vi "MasterControl.vi"() -> ()   [LabVIEW 2012]
uses:
  VI State Control.ctl
  TMC/Set Parameter.ctl
  LabView VI's/Source Mirror Manipulator/Axis.ctl
  SMC VIs - Pollux/SMC SubVIs/SMC_SubVIs.llb/SMC Paras.ctl
  SMC VIs - Pollux/SMC SubVIs/SMC_SubVIs.llb/VENUSNr.ctl
  SMC VIs - Pollux/SubVIs/JS_Comm.llb/Comm_Paras.ctl
  SMC VIs - Pollux/SubVIs/JS_Comm.llb/Comm_Method.ctl
panel:
  out "Diode 1":string
  out "Diode 3":string
  out "Diode 2":string
  in  "Time Delay":u32
  in  "File Path for Data Log":path=path "C:/Users/user/Desktop/labviewMove/stats/stats_00-00-00.txt"
  out "Error":bool
  out "VI Status":bool
  in  "Anode Control":enum16{"1", "2", "3", "4", "5", "6"}(ring)
  out "Axis Information":string
  in  "Axis Positions":T1
  out "VI State Control":T2
  out "Source Mirror Position (mm)":dbl(slide) scale=0.0..50.0 scale format="%#.6g"
  in  "Voltage Value":dbl
  in  "Set Source Voltage":bool
  out "Current (mA)":dbl
  out "Source Voltage":dbl
  out "Logging Indicator":bool
  in  "Source Voltage Control":bool
  out "Limit A":bool
  out "Limit B":bool
  out "Home":bool
  in  "Main Axis Control":T3(ring)
  out "Anode :":u32(knob) scale=1.0..6.0
  in  "Target":dbl
  out "Current Position:":dbl
  in  "Absolute Position Value":dbl
  in  "Index +/- Value":dbl
  in  "Stop Program":bool
  in  "Abort Motion":bool
  in  "Stop Motion Softly":bool
  in  "Move to Absolute Positon":bool
  in  "Position Index +/-":bool
  in  "Reset Position to Target":bool
  in  "Go To Home Position":bool
  # "--  Master Control  --"
  # "sec"
  # "Data Logging Control"
  # "Keep file type as a '.txt' file"
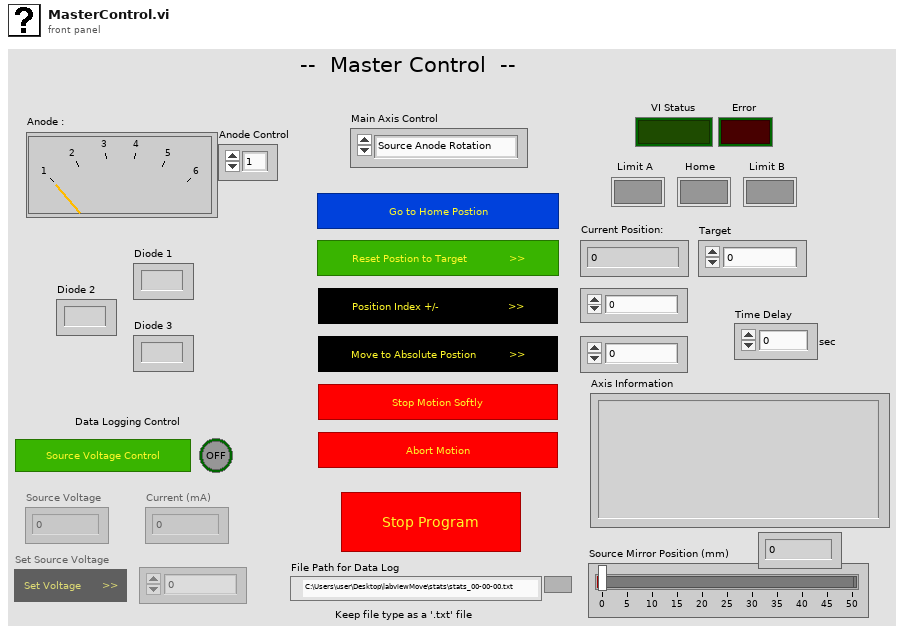
[diagram p1: front panel]
types:
  T1 = cluster{"Source Anode Rotation (P)":dbl, "Aperture Translation (P)":dbl, "Grating Translation (P)":dbl, "Grating Vertical (P)":dbl, "Grating Rotation (P)":dbl, "Polarization Angle (P)":dbl, "Source Mirror Translation (P)":dbl, "Source Mirror Rotation (P)":dbl, "Camera Translation (P)":dbl, "Camera Vertical (P) ":dbl, "Detector Mirror Rotation (P)":dbl}
  T2 = typedef "VI State Control.ctl" = enum16{"Initialization", "Wait for Command", "Add New State Here"}
  T3 = enum16{"Source Anode Rotation", "Aperture Translation", "Grating Translation", "Grating Vertical", "Grating Rotation", "Polarization Angle", "Source Mirror Translation", "Source Mirror Rotation", "Camera Translation", "Camera Vertical", "Detector Mirror Rotation"}
  T4 = enum16{"open", "replace", "create", "open or create", "replace or create", "replace or create with confirmation"}
  T5 = typedef "Axis.ctl" = enum16{"Translation", "Rotation"}
  T6 = typedef "Set Parameter.ctl" = enum16{"Acceleration (A)", "Baud Rate (BD)", "Counter 1 (C1)", "Counter 2 (C2)", "Control C Software Reset (CE)", "Check Sum Enable (CK)", "Clock Mode (CM)", "Clock Mode Ratio (CR)", "Clock Mode Out Step Width (CW)", "Deceleration (D)", "Digital Filtering, Input 1 (D1)", "Digital Filtering, Input 2 (D2)", "Digital Filtering, Input 3 (D3)", "Digital Filtering, Input 4 (D4)", "Digital Filtering, Input 5 (D5)", "Digital Filtering, Input 9 (D9)", "Digital Filtering, Input 10 (D10)", "Digital Filtering, Input 11 (D11)", "Digital Filtering, Input 12 (D12)", "Deadband (DB)", "Decrement Variable (DC)", "Enable/Disable Drive (DE)", "Device Name (DN)", "End Program Execution (E)", "Encoder Function Enable (EE)", "Encoder Lines (EL)", "Echo Mode (EM)", "Escape (ES)", "Execute Program at Address (EX)", "Hold (H)", "Hold Current (HC)", "Hold Current Delay Time (HI)", "Home to Encoder Index (HM)", "Home to Home Switch (HT)", "Increment Variable (IC)", "Initialize Parameters to NVM (IP)", "Input into Variable (IV)", "Jog Enable (JE)", "Limit Stop Mode (LM)", "Move Absolute (MA)", "Move Relative (MR)", "MicroStepping Select (MS)", "Motor Settling Delay Time (MT)", "Output 1 (O1)", "Output 2 (O2)", "Output 3 (O3)", "Output 4 (O4)", "Output 9 (O9)", "Output 10 (O10)", "Output 11 (O11)", "Output 12 (O12)", "Output High Byte (9-12) (OH)", "Output Low Byte (1-4) (OL)", "Output Total (1-4 and 9-12) (OT)", "Position Maintenance (PM)", "Party Mode (PY)", "Register 1 (R1)", "Register 2 (R2)", "Register 3 (R3)", "Register 4 (R4)", "Run Current (RC)", "Stall Factor (SF)", "Slew (SL)", "Stall Mode Set (SM)", "Upgrade Firmware (UG)", "Velocity Initial (VI)", "Velocity Maximum (VM)"}
  T7 = typedef "Comm_Paras.ctl" = cluster{"Comm Method":T8, "IP Address":string, "Remote Port":u16, "GPIB Address":string, "VISA Resource Name":refnum<visa-resource-name>, "Visa Baud Rate":u32, "Visa Serial":bool}
  T8 = typedef "Comm_Method.ctl" = enum16{"TCPIP", "GPIB", "VISA"}
  T9 = typedef "SMC Paras.ctl" = cluster{"VENUS Language":T10, "Number of Axis":u8, "Controller Nr":u8, "Simulation":bool}
  T10 = typedef "VENUSNr.ctl" = enum16{"VENUS 2", "VENUS 1"}
  T11 = enum8{"Enabled", "Disabled", "Disabled and Grayed Out"}
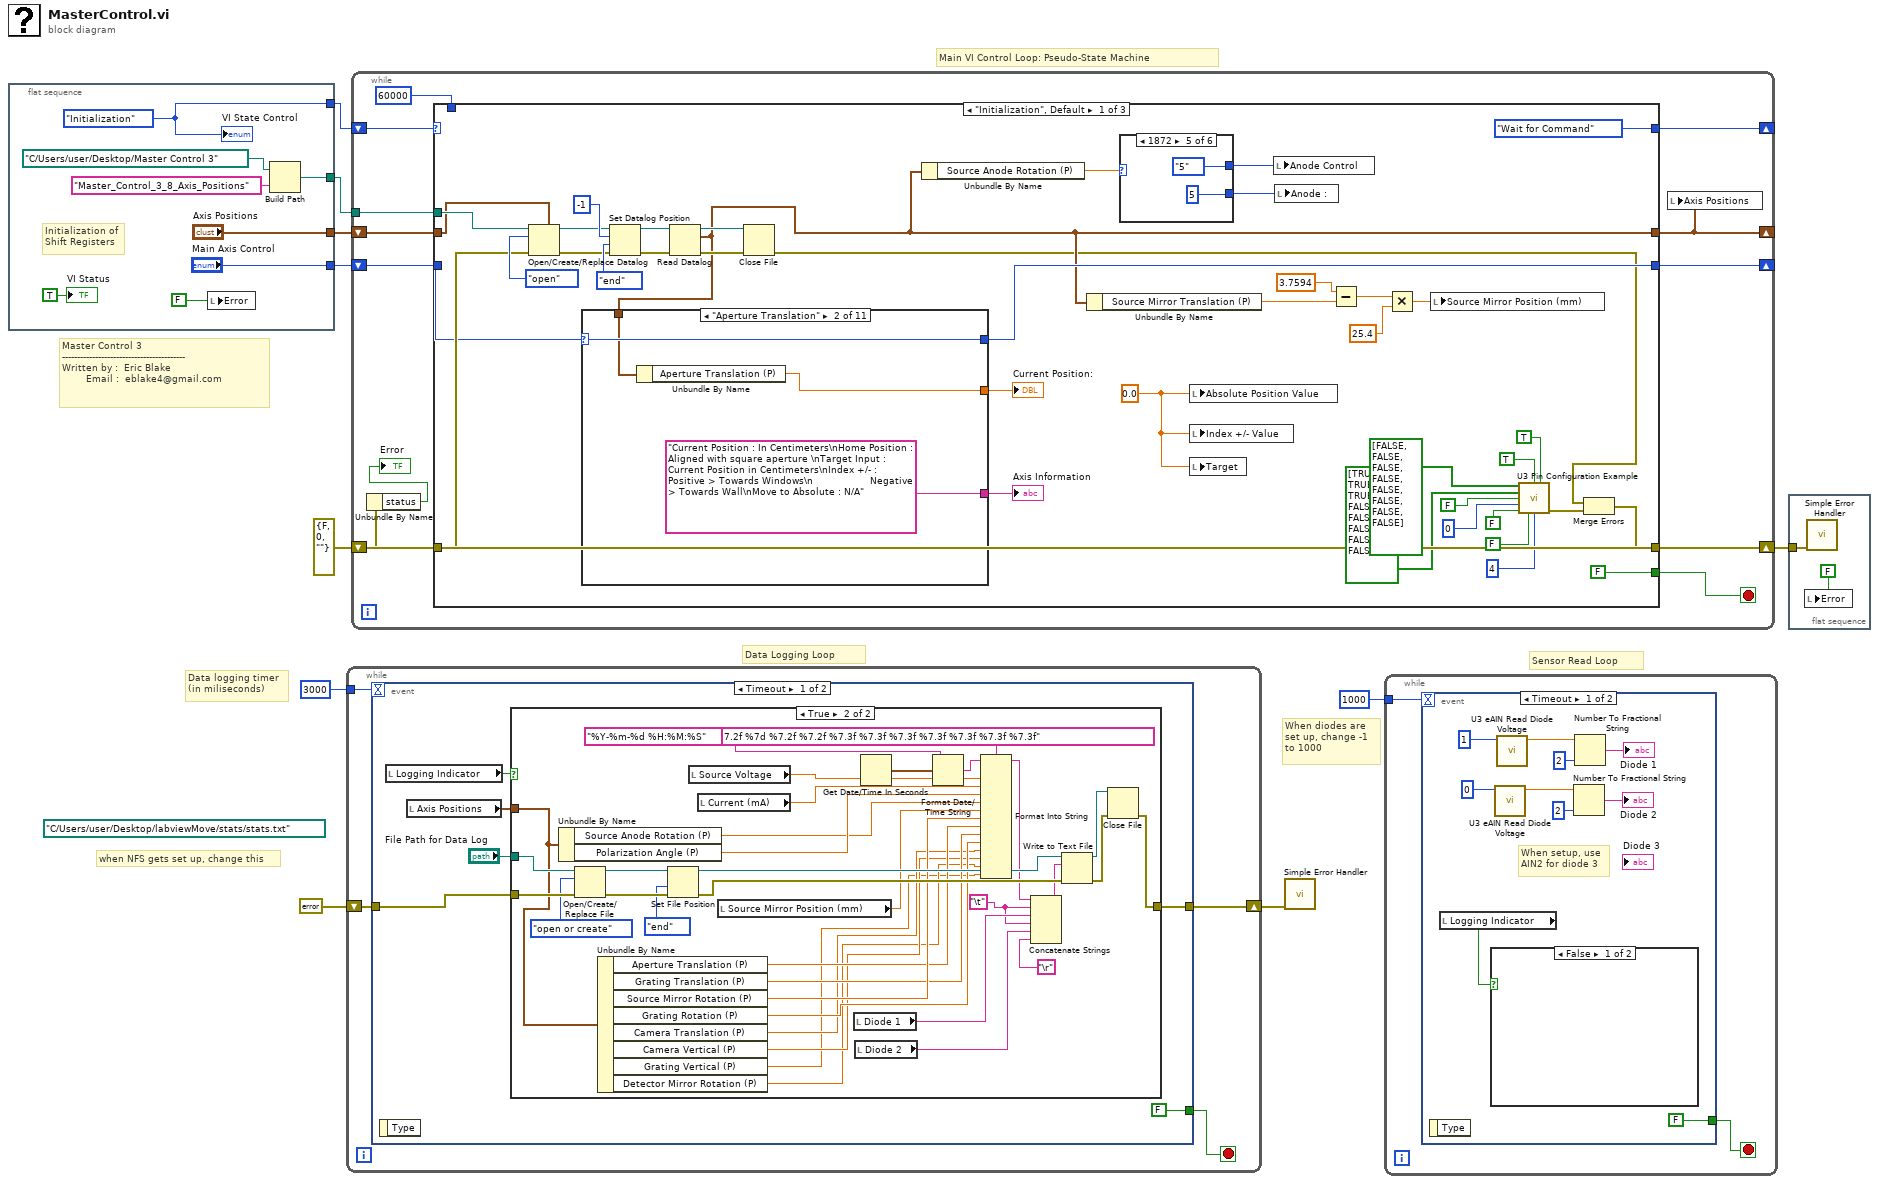
[diagram p0: block diagram]
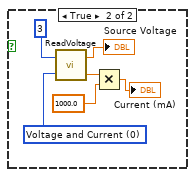
[diagram p2: hidden frame]
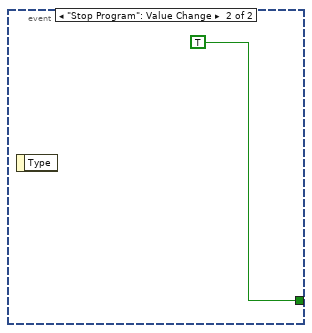
[diagram p3: hidden frame]
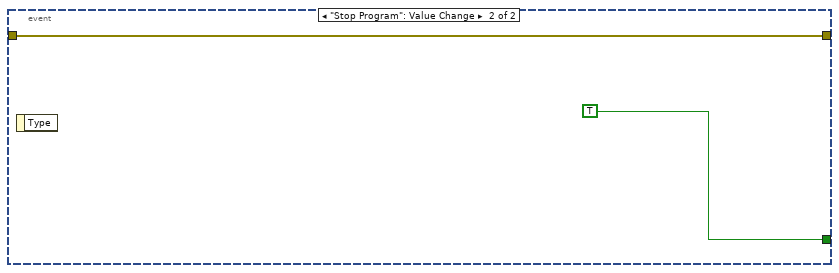
[diagram p5: hidden frame]
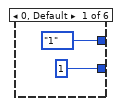
[diagram p6: hidden frame]
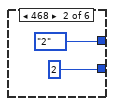
[diagram p7: hidden frame]
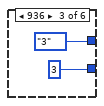
[diagram p8: hidden frame]
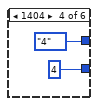
[diagram p9: hidden frame]
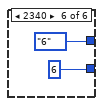
[diagram p10: hidden frame]
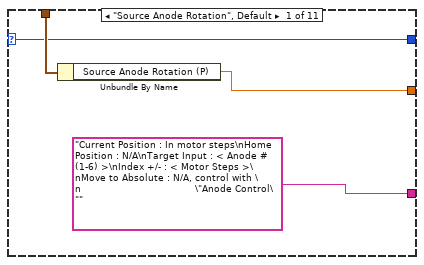
[diagram p11: hidden frame]
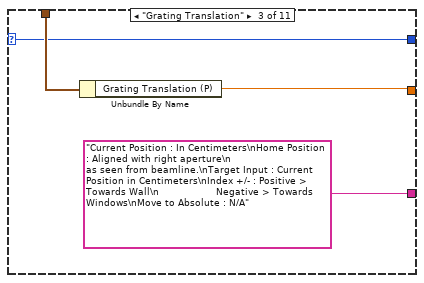
[diagram p12: hidden frame]
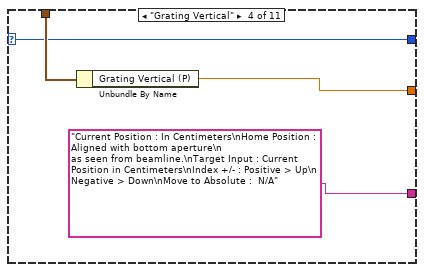
[diagram p13: hidden frame]
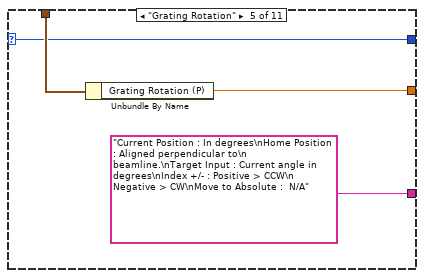
[diagram p14: hidden frame]
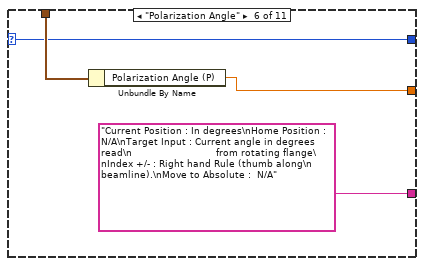
[diagram p15: hidden frame]
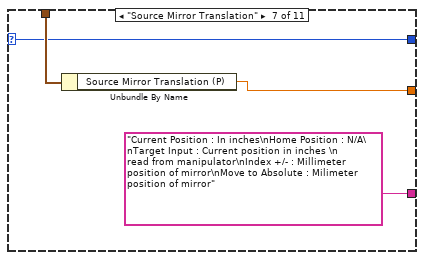
[diagram p16: hidden frame]
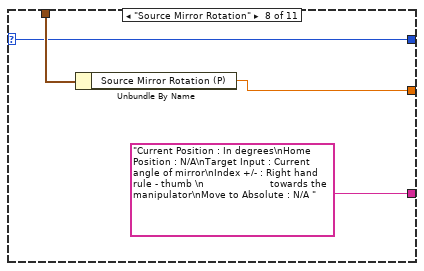
[diagram p17: hidden frame]
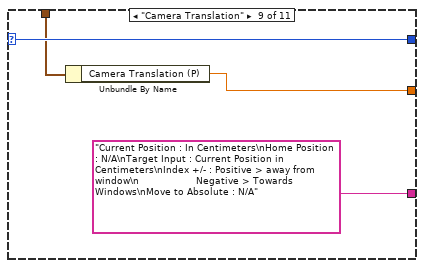
[diagram p18: hidden frame]
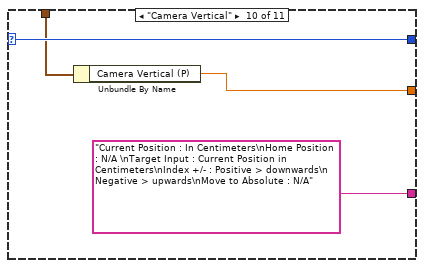
[diagram p19: hidden frame]
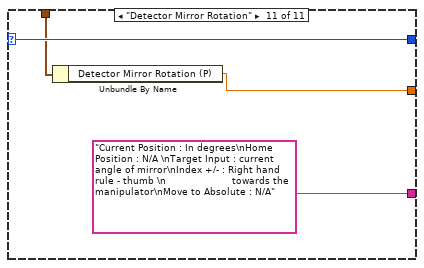
[diagram p20: hidden frame]
diagram:
  (unwired) path "C:/Users/user/Desktop/labviewMove/stats/stats.txt" ("file path (use dialog)")
  # "Master Control 3\n-----------------------------------------\nWritten by :  Eric Blake\n        Email :  eblake4@gmail.com"
  # "when NFS gets set up, change this"
  # "When diodes are \nset up, change -1 \nto 1000"
  # "Sensor Read Loop"
  # "Main VI Control Loop: Pseudo-State Machine"
  # "Data Logging Loop"
  # "Data logging timer\n(in miliseconds)"
  n1 = flat-sequence {
    tunnel: [w18] -> w10
    tunnel: [w15] -> w8
    tunnel: ["Main Axis Control"] -> w7
    tunnel: ["Axis Positions"] -> w6
    frame #0 {
      w18 = VI_State_Control."Initialization" ("VI State Control")
      # "Initialization of\nShift Registers"
      n2 = local write "Error"(FALSE) -> ()
      n3 = Build Path(base path=path "C:/Users/user/Desktop/Master Control 3", name or relative path="Master_Control_3_8_Axis_Positions") -> (appended path=w15:path)
      "VI State Control" <- w18
      "VI Status" <- TRUE ("VI on")
    }
  }
  n4 = while {
    tunnel: 3000 -> [w22]
    shift-right: [w19] -> w3
    shift-left: errorcluster {"status"=FALSE, "code"=0, "source"=""} ("error out") -> [w20]
    stop <- w21 stop-if-true
    n5 = event shown="[0] Timeout" {
      selector: _ -> [_ _]
      dyn-events: _ -> [_ _]
      timeout: w22 -> [_ _]
      tunnel: [FALSE TRUE] -> w21
      tunnel: [w25 w65] -> w19
      tunnel: w20 -> [w24 w65]
      event Timeout {
        n6 = event-data() -> ()  [unwired: 1 in, 1 out]
        n7 = local read "Logging Indicator"() -> (w26:bool)
        n8 = local read "Axis Positions"() -> (w27:T1)
        n9 = case shown="True" w26 {
          tunnel: w27 -> [_ w45]
          tunnel: [w29 w52] -> w25
          tunnel: w24 -> [w29 w51]
          tunnel: "File Path for Data Log" -> [_ w48]
          frame False {
          }
          frame True {
            w36 = "\t"
            n10 = Unbundle By Name(w45) -> ("Source Anode Rotation (P)"=w53:dbl, "Polarization Angle (P)"=w57:dbl)
            n11 = Open/Create/Replace File(file path (use dialog)=w48, error in=w51, operation (0:open)=T4."open or create") -> (refnum out=w63:refnum<file>, error out=w64:errorcluster)  [unwired: 4 out]
            n12 = Unbundle By Name(w45) -> ("Aperture Translation (P)"=w42:dbl, "Grating Translation (P)"=w41:dbl, "Source Mirror Rotation (P)"=w43:dbl, "Grating Rotation (P)"=w34:dbl, "Camera Translation (P)"=w33:dbl, "Camera Vertical (P)"=w32:dbl, "Grating Vertical (P)"=w30:dbl, "Detector Mirror Rotation (P)"=w31:dbl)
            n13 = Set File Position(refnum=w63, from (0:start)=enum16{"start", "end", "current"}."end", error in=w64) -> (refnum out=w56:refnum<file>, error out=w50:errorcluster)  [unwired: 1 out]
            n14 = local read "Source Voltage"() -> (w46:dbl)
            n15 = local read "Current (mA)"() -> (w47:dbl)
            n16 = local read "Source Mirror Position (mm)"() -> (w49:dbl)
            n17 = local read "Diode 1"() -> (w37:string)
            n18 = local read "Diode 2"() -> (w35:string)
            n19 = Get Date/Time In Seconds() -> (seconds since 1Jan1904=w61:timestamp)
            n20 = Format Date/Time String(time format string (%c)="%Y-%m-%d %H:%M:%S", seconds (now)=w61) -> (date/time string=w59:string)  [unwired: 1 out]
            n21 = Format Into String(format string=" %7.1f %7.4f %+7.2f %7d %7.2f %7.2f %7.3f %7.3f %7.3f %7.3f %7.3f %7.3f %7.3f", initial string=w59, w46, w47, w57, w53, w49, w43, w42, w41, w34, w33, w32, w31, w30) -> (resulting string=w40:string)  [unwired: 1 in, 1 out]
            n22 = Concatenate Strings(w40, w36, w37, w36, w35, "\r") -> (w39:string)
            n23 = Write to Text File(file (use dialog)=w56, text=w39, error in=w50) -> (refnum out=w55:refnum<file>, error out=w54:errorcluster)  [unwired: 2 out]
            n24 = Close File(refnum=w55, error in=w54) -> (error out=w52:errorcluster)  [unwired: 1 out]
          }
        }
      }
      event "Stop Program": Value Change {
        n25 = event-data() -> ()  [unwired: 1 in, 1 out]
      }
    }
  }
  n26 = while {
    tunnel: w8 -> [w76]
    shift-right: [w77] -> _
    shift-left: w10 -> [w78]
    shift-right: [w69] -> w9
    shift-left: errorcluster {"status"=FALSE, "code"=0, "source"=""} ("error out") -> [w75]
    shift-right: [w74] -> _
    shift-left: w7 -> [w73]
    shift-right: [w71] -> _
    shift-left: w6 -> [w72]
    stop <- w70 stop-if-true
    n27 = case shown="\"Initialization\", Default" w78 {
      tunnel: [FALSE w184 FALSE] -> w70
      tunnel: [VI_State_Control."Wait for Command" ("VI State Control") w183 VI_State_Control."Wait for Command" ("VI State Control")] -> w77
      tunnel: w76 -> [w112 w180 _]
      tunnel: [w80 w181 w1061] -> w69
      tunnel: w75 -> [w107 w182 w1061]
      tunnel: [w105 w179 w1064] -> w74
      tunnel: w73 -> [w103 w178 w1064]
      tunnel: w72 -> [w104 w177 w1065]
      tunnel: [w96 w176 w1065] -> w71
      tunnel: 60000 -> [_ w175 _]
      frame "Initialization", Default {
        w94 = 0.0 ("Absolute Position Value")
        n28 = Open/Create/Replace Datalog(5:w104, 8:w107, 10:T4."open" ("operation (0:open)"), 11:w112) -> (0:w110:errorcluster, 3:w111:refnum<k1>)  [unwired: 2 in, 1 out]
        n29 = Set Datalog Position(4:w110, 5:enum16{"start", "end", "current"}."end" ("from (0:start)"), 6:i64 -1 ("offset (in records) (0)"), 7:w111) -> (0:w109:errorcluster, 3:w116:refnum<k1>)
        n30 = Read Datalog(4:w109, 7:w116) -> (0:w108:errorcluster, 2:w96:T1, 3:w117:refnum<k1>)  [unwired: 1 in]
        n31 = case shown="\"Aperture Translation\"" w103 {
          selector: w103 -> [w133 w138 w141 w145 w149 w153 w157 w161 w166 w170 w174]
          tunnel: [w133 w138 w141 w145 w149 w153 w157 w161 w166 w170 w174] -> w105
          tunnel: w96 -> [w134 w137 w142 w146 w150 w154 w158 w162 w165 w169 w173]
          tunnel: [w132 w136 w140 w144 w148 w152 w156 w160 w164 w168 w172] -> w101
          tunnel: ["Current Position : In motor steps\nHome Position : N/A\nTarget Input : < Anode # (1-6) >\nIndex +/- : < Motor Steps >\nMove to Absolute : N/A, control with \n                                      \"Anode Control\"" "Current Position : In Centimeters\nHome Position : Aligned with square aperture \nTarget Input : Current Position in Centimeters\nIndex +/- : Positive > Towards Windows\n                   Negative > Towards Wall\nMove to Absolute : N/A" "Current Position : In Centimeters\nHome Position : Aligned with right aperture\n                              as seen from beamline.\nTarget Input : Current Position in Centimeters\nIndex +/- : Positive > Towards Wall\n                   Negative > Towards Windows\nMove to Absolute : N/A" "Current Position : In Centimeters\nHome Position : Aligned with bottom aperture\n                              as seen from beamline.\nTarget Input : Current Position in Centimeters\nIndex +/- : Positive > Up\n                   Negative > Down\nMove to Absolute :  N/A" "Current Position : In degrees\nHome Position : Aligned perpendicular to\n                                beamline.\nTarget Input : Current angle in degrees\nIndex +/- : Positive > CCW\n                   Negative > CW\nMove to Absolute :  N/A" "Current Position : In degrees\nHome Position : N/A\nTarget Input : Current angle in degrees read\n                            from rotating flange\nIndex +/- : Right hand Rule (thumb along\n                       beamline).\nMove to Absolute :  N/A" "Current Position : In inches\nHome Position : N/A\nTarget Input : Current position in inches \n                           read from manipulator\nIndex +/- : Millimeter position of mirror\nMove to Absolute : Milimeter position of mirror" "Current Position : In degrees\nHome Position : N/A\nTarget Input : Current angle of mirror\nIndex +/- : Right hand rule - thumb \n                      towards the manipulator\nMove to Absolute : N/A " "Current Position : In Centimeters\nHome Position : N/A\nTarget Input : Current Position in Centimeters\nIndex +/- : Positive > away from window\n                   Negative > Towards Windows\nMove to Absolute : N/A" "Current Position : In Centimeters\nHome Position : N/A \nTarget Input : Current Position in Centimeters\nIndex +/- : Positive > downwards\n                   Negative > upwards\nMove to Absolute : N/A" "Current Position : In degrees\nHome Position : N/A \nTarget Input : current angle of mirror\nIndex +/- : Right hand rule - thumb \n                      towards the manipulator\nMove to Absolute : N/A"] -> w102
          frame "Source Anode Rotation", Default {
            n32 = Unbundle By Name(w134) -> ("Source Anode Rotation (P)"=w132:dbl)
          }
          frame "Aperture Translation" {
            n33 = Unbundle By Name(w137) -> ("Aperture Translation (P)"=w136:dbl)
          }
          frame "Grating Translation" {
            n34 = Unbundle By Name(w142) -> ("Grating Translation (P)"=w140:dbl)
          }
          frame "Grating Vertical" {
            n35 = Unbundle By Name(w146) -> ("Grating Vertical (P)"=w144:dbl)
          }
          frame "Grating Rotation" {
            n36 = Unbundle By Name(w150) -> ("Grating Rotation (P)"=w148:dbl)
          }
          frame "Polarization Angle" {
            n37 = Unbundle By Name(w154) -> ("Polarization Angle (P)"=w152:dbl)
          }
          frame "Source Mirror Translation" {
            n38 = Unbundle By Name(w158) -> ("Source Mirror Translation (P)"=w156:dbl)
          }
          frame "Source Mirror Rotation" {
            n39 = Unbundle By Name(w162) -> ("Source Mirror Rotation (P)"=w160:dbl)
          }
          frame "Camera Translation" {
            n40 = Unbundle By Name(w165) -> ("Camera Translation (P)"=w164:dbl)
          }
          frame "Camera Vertical" {
            n41 = Unbundle By Name(w169) -> ("Camera Vertical (P)"=w168:dbl)
          }
          frame "Detector Mirror Rotation" {
            n42 = Unbundle By Name(w173) -> ("Detector Mirror Rotation (P)"=w172:dbl)
          }
        }
        "Axis Information" <- w102
        "Current Position:" <- w101
        n43 = Close File(refnum=w117, error in=w108) -> (error out=w81:errorcluster)  [unwired: 1 out]
        n44 = Unbundle By Name(w96) -> ("Source Anode Rotation (P)"=w100:dbl)
        n45 = Unbundle By Name(w96) -> ("Source Mirror Translation (P)"=w95:dbl)
        n46 = case shown="1872" w100 {
          tunnel: [enum16{"1", "2", "3", "4", "5", "6"}."1" ("Anode Control") enum16{"1", "2", "3", "4", "5", "6"}."2" ("Anode Control") enum16{"1", "2", "3", "4", "5", "6"}."3" ("Anode Control") enum16{"1", "2", "3", "4", "5", "6"}."4" ("Anode Control") enum16{"1", "2", "3", "4", "5", "6"}."5" ("Anode Control") enum16{"1", "2", "3", "4", "5", "6"}."6" ("Anode Control")] -> w98
          tunnel: [u32 1 ("Anode :") u32 2 ("Anode :") u32 3 ("Anode :") u32 4 ("Anode :") u32 5 ("Anode :") u32 6 ("Anode :")] -> w99
          frame 0, Default {
          }
          frame 468 {
          }
          frame 936 {
          }
          frame 1404 {
          }
          frame 1872 {
          }
          frame 2340 {
          }
        }
        n47 = local write "Absolute Position Value"(w94) -> ()
        n48 = local write "Index +/- Value"(w94) -> ()
        n49 = local write "Target"(w94) -> ()
        n50 = local write "Anode Control"(w98) -> ()
        n51 = local write "Anode :"(w99) -> ()
        n52 = Subtract(x=3.7594, y=w95) -> (x-y=w92:dbl)
        n53 = Multiply(x=w92, y=25.4) -> (x*y=w91:dbl)
        n54 = local write "Source Mirror Position (mm)"(w91) -> ()
        n55 = call "U3 Pin Configuration Example.vi"("FIO Analog Enable"=bool[] [FALSE, FALSE, FALSE, FALSE, FALSE, FALSE, FALSE, FALSE], "FirstFound"=TRUE, "Set Defaults"=TRUE, "EIO Analog Enable"=bool[] [TRUE, TRUE, TRUE, FALSE, FALSE, FALSE, FALSE, FALSE], "Enable DAC1"=FALSE, "Number of Timers Enabled"=u8 0, "Enable Counter0"=FALSE, "Enable Counter1"=FALSE, "Timer/Counter Pin Offset"=u8 4) -> ("error out"=w79:errorcluster)  [unwired: 5 in, 1 out]
        n56 = Merge Errors(w81, w79) -> (w80:errorcluster)
      }
      frame "Wait for Command" {
        n57 = event shown="[5] \"Position Index +/-\": Value Change" {
          selector: _ -> [_ _ _ _ _ _ _ _ _ _ _ _]
          dyn-events: _ -> [_ _ _ _ _ _ _ _ _ _ _ _]
          timeout: w175 -> [_ _ _ _ _ _ _ _ _ _ _ _]
          tunnel: [FALSE TRUE FALSE FALSE FALSE FALSE FALSE FALSE FALSE FALSE FALSE FALSE] -> w184
          tunnel: [VI_State_Control."Wait for Command" ("VI State Control") VI_State_Control."Wait for Command" ("VI State Control") VI_State_Control."Wait for Command" ("VI State Control") VI_State_Control."Wait for Command" ("VI State Control") VI_State_Control."Wait for Command" ("VI State Control") VI_State_Control."Wait for Command" ("VI State Control") VI_State_Control."Wait for Command" ("VI State Control") VI_State_Control."Wait for Command" ("VI State Control") VI_State_Control."Wait for Command" ("VI State Control") VI_State_Control."Wait for Command" ("VI State Control") VI_State_Control."Wait for Command" ("VI State Control") VI_State_Control."Wait for Command" ("VI State Control")] -> w183
          tunnel: w182 -> [w190 w210 w226 w288 w422 w520 w813 w900 w968 w1031 w1038 w1055]
          tunnel: [w188 w206 w225 w287 w424 w528 w820 w905 w969 w1031 w1038 w1055] -> w181
          tunnel: w180 -> [w191 w211 _ _ _ _ _ _ _ _ _ _]
          tunnel: [w197 w204 w224 w292 w426 w525 w819 w903 w967 w1033 w1037 w1054] -> w179
          tunnel: w178 -> [w197 w204 _ w292 w429 w527 w819 w906 w967 w1033 w1037 w1054]
          tunnel: w177 -> [w185 w202 w220 w291 w428 w521 w817 w902 w972 w1032 w1036 w1053]
          tunnel: [w185 w202 w220 w290 w425 w526 w816 w901 w970 w1032 w1036 w1053] -> w176
          event Timeout {
            n58 = event-data() -> ()  [unwired: 1 in, 1 out]
            n59 = Open/Create/Replace Datalog(5:w185, 8:w190, 10:T4."open or create" ("operation (0:open)"), 11:w191) -> (0:w194:errorcluster, 3:w187:refnum<k1>)  [unwired: 2 in, 1 out]
            n60 = Set Datalog Position(4:w194, 5:enum16{"start", "end", "current"}."end" ("from (0:start)"), 7:w187) -> (0:w193:errorcluster, 3:w186:refnum<k1>)  [unwired: 1 in]
            n61 = Write Datalog(4:w193, 6:w185, 7:w186) -> (0:w192:errorcluster, 3:w189:refnum<k1>)
            n62 = Close File(refnum=w189, error in=w192) -> (error out=w188:errorcluster)  [unwired: 1 out]
          }
          event "Stop Program": Value Change {
            w200 = T11."Disabled and Grayed Out" ("Disabled")
            w201 = FALSE
            n63 = event-data() -> ()  [unwired: 1 in, 1 out]
            n64 = Open/Create/Replace Datalog(5:w202, 8:w210, 10:T4."open or create" ("operation (0:open)"), 11:w211) -> (0:w209:errorcluster, 3:w215:refnum<k1>)  [unwired: 2 in, 1 out]
            n65 = Set Datalog Position(4:w209, 5:enum16{"start", "end", "current"}."end" ("from (0:start)"), 7:w215) -> (0:w208:errorcluster, 3:w214:refnum<k1>)  [unwired: 1 in]
            n66 = local write "VI Status"(w201) -> ()
            n67 = local write "Home"(w201) -> ()
            n68 = local write "Limit A"(w201) -> ()
            n69 = local write "Limit B"(w201) -> ()
            n70 = local write "Error"(w201) -> ()
            n71 = local write "Logging Indicator"(w201) -> ()
            n72 = Write Datalog(4:w208, 6:w202, 7:w214) -> (0:w207:errorcluster, 3:w212:refnum<k1>)
            n73 = Close File(refnum=w212, error in=w207) -> (error out=w206:errorcluster)  [unwired: 1 out]
            n74 = property on="Source Voltage" class="DigNum (strict)"("DisabledEnum"=w200) -> ()  [unwired: 2 in, 2 out]
            n75 = property on="Current (mA)" class="DigNum (strict)"("DisabledEnum"=w200) -> ()  [unwired: 2 in, 2 out]
            n76 = property on="Set Source Voltage" class="Bool"("DisabledEnum"=w200) -> ()  [unwired: 2 in, 2 out]
            n77 = property on="Voltage Value" class="DigNum (strict)"("DisabledEnum"=w200) -> ()  [unwired: 2 in, 2 out]
          }
          event "Main Axis Control": Value Change {
            w219 = 0.0 ("Index +/- Value")
            n78 = event-data() -> ()  [unwired: 1 in, 1 out]
            n79 = local read "Main Axis Control"() -> (w223:T3)
            n80 = case shown="\"Camera Vertical\"" w223 {
              selector: w223 -> [w232 w237 w242 w245 w252 w257 w262 w267 w272 w277 w282]
              tunnel: w220 -> [w234 w239 w244 w249 w254 w259 w264 w269 w274 w279 w284]
              tunnel: [w233 w238 w243 w248 w253 w258 w263 w268 w273 w278 w283] -> w225
              tunnel: w226 -> [w233 w238 w243 w248 w253 w258 w263 w268 w273 w278 w283]
              tunnel: [w232 w237 w242 w245 w252 w257 w262 w267 w272 w277 w282] -> w224
              tunnel: ["Current Position : In motor steps\nHome Position : N/A\nTarget Input : < Anode # (1-6) >\nIndex +/- : < Motor Steps >\nMove to Absolute : N/A, control with \n                                      \"Anode Control\"" "Current Position : In Centimeters\nHome Position : Aligned with square aperture \nTarget Input : Current Position in Centimeters\nIndex +/- : Positive > Towards Wall\n                   Negative > Towards Windows\nMove to Absolute : N/A" "Current Position : In Centimeters\nHome Position : Aligned with right aperture\n                              as seen from beamline.\nTarget Input : Current Position in Centimeters\nIndex +/- : Positive > Towards Wall\n                   Negative > Towards Windows\nMove to Absolute : N/A" "Current Position : In Centimeters\nHome Position : Aligned with bottom aperture\n                              as seen from beamline.\nTarget Input : Current Position in Centimeters\nIndex +/- : Positive > Down\n                   Negative > Up\nMove to Absolute :  N/A" "Current Position : In degrees\nHome Position : Aligned perpendicular to\n                                beamline.\nTarget Input : Current angle in degrees\nIndex +/- : Positive > CCW\n                   Negative > CW\nMove to Absolute :  N/A" "Current Position : In degrees\nHome Position : N/A\nTarget Input : Current angle in degrees read\n                            from rotating flange\nIndex +/- : Right hand Rule (thumb along\n                       beamline).\nMove to Absolute :  N/A" "Current Position : In inches\nHome Position : N/A\nTarget Input : Current position in inches \n                           read from manipulator\nIndex +/- : Millimeter position of mirror\nMove to Absolute : Milimeter position of mirror" "Current Position : In degrees\nHome Position : N/A\nTarget Input : Current angle of mirror\nIndex +/- : Right hand rule - thumb \n                      towards the manipulator\nMove to Absolute : N/A " "Current Position : In Centimeters\nHome Position : N/A \nTarget Input : Current Position in Centimeters\nIndex +/- : Positive > away from window\n                   Negative > Towards Windows\nMove to Absolute : N/A" "Current Position : In Centimeters\nHome Position : N/A \nTarget Input : Current Position in Centimeters\nIndex +/- : Positive >  downwards\n                   Negative > upwards \nMove to Absolute : N/A" "Current Position : In degrees\nHome Position :  N/A \nTarget Input : Current angle of mirror\nIndex +/- : Right Hand Rule - thumb \n                    towards the manipulator\nMove to Absolute : N/A"] -> w222
              tunnel: [w231 w235 w240 w247 w251 w256 w261 w266 w270 w275 w280] -> w218
              frame "Source Anode Rotation", Default {
                n81 = Unbundle By Name(w234) -> ("Source Anode Rotation (P)"=w231:dbl)
              }
              frame "Aperture Translation" {
                n82 = Unbundle By Name(w239) -> ("Aperture Translation (P)"=w235:dbl)
              }
              frame "Grating Translation" {
                n83 = Unbundle By Name(w244) -> ("Grating Translation (P)"=w240:dbl)
              }
              frame "Grating Vertical" {
                n84 = Unbundle By Name(w249) -> ("Grating Vertical (P)"=w247:dbl)
              }
              frame "Grating Rotation" {
                n85 = Unbundle By Name(w254) -> ("Grating Rotation (P)"=w251:dbl)
              }
              frame "Polarization Angle" {
                n86 = Unbundle By Name(w259) -> ("Polarization Angle (P)"=w256:dbl)
              }
              frame "Source Mirror Translation" {
                n87 = Unbundle By Name(w264) -> ("Source Mirror Translation (P)"=w261:dbl)
              }
              frame "Source Mirror Rotation" {
                n88 = Unbundle By Name(w269) -> ("Source Mirror Rotation (P)"=w266:dbl)
              }
              frame "Camera Translation" {
                n89 = Unbundle By Name(w274) -> ("Camera Translation (P)"=w270:dbl)
              }
              frame "Camera Vertical" {
                n90 = Unbundle By Name(w279) -> ("Camera Vertical (P)"=w275:dbl)
              }
              frame "Detector Mirror Rotation" {
                n91 = Unbundle By Name(w284) -> ("Detector Mirror Rotation (P)"=w280:dbl)
              }
            }
            n92 = local write "Axis Information"(w222) -> ()
            n93 = local write "Current Position:"(w218) -> ()
            n94 = Equal To 0?(x=w218) -> (x = 0?=w217:bool)
            n95 = local write "Index +/- Value"(w219) -> ()
            n96 = local write "Absolute Position Value"(w219) -> ()
            n97 = local write "Target"(w219) -> ()
            n98 = case shown="True" w217 {
              selector: w217 -> [w228 w229]
              frame False {
                n99 = local write "Home"(w228) -> ()
              }
              frame True {
                n100 = local write "Home"(w229) -> ()
              }
            }
          }
          event "Go To Home Position": Value Change {
            n101 = event-data() -> ()  [unwired: 1 in, 1 out]
            n102 = case shown="\"Camera Vertical\"" w292 {
              tunnel: w291 -> [w299 w303 w329 w351 w372 w396 w401 w406 w411 w416 w421]
              tunnel: [w299 w304 w328 w352 w371 w396 w401 w406 w411 w416 w421] -> w290
              tunnel: w288 -> [w301 w313 w335 w354 w376 w395 w400 w405 w410 w415 w420]
              tunnel: [w301 w305 w330 w349 w373 w395 w400 w405 w410 w415 w420] -> w289
              tunnel: [w300 w302 w327 w350 w370 w393 w399 w403 w408 w413 w418] -> w286
              tunnel: [FALSE TRUE TRUE TRUE TRUE FALSE FALSE FALSE FALSE FALSE FALSE] -> w285
              frame "Source Anode Rotation", Default {
                n103 = One Button Dialog(message="No Home Position\nSet for this Axis.") -> ()  [unwired: 1 in, 1 out]
                n104 = local read "Current Position:"() -> (w300:dbl)
              }
              frame "Aperture Translation" {
                w308 = refnum<visa-resource-name> "COM8" ("VISA resource name IN")
                w309 = "G" ("Axis Prefix")
                n105 = call "AMS Move Motor.vi"("error in"=w313, "Motor steps"=-200000.0, "Axis Prefix"=w309, "VISA resource name IN"=w308) -> ("error out"=w310:errorcluster)  [unwired: 6 in, 1 out]
                n106 = call "AMS Move Motor.vi"("error in"=w310, "Motor steps"=9680.0, "Axis Prefix"=w309, "VISA resource name IN"=w308) -> ("error out"=w311:errorcluster)  [unwired: 6 in, 1 out]
                n107 = flat-sequence {
                  tunnel: [w322] -> w306
                  tunnel: w311 -> [w322]
                  frame #0 {
                    n108 = Wait (ms)(milliseconds to wait=u32 50000) -> ()  [unwired: 1 out]
                  }
                }
                n109 = case shown="No Error" w306 {
                  selector: w306 -> [w318 w320]
                  tunnel: [w318 w320] -> w305
                  tunnel: w303 -> [w317 w321]
                  tunnel: [w316 w321] -> w304
                  tunnel: [w315 w319] -> w302
                  frame No Error {
                    w315 = 0.0 ("Source Anode Rotation (P)")
                    n110 = Bundle By Name(cluster=w317, "Aperture Translation (P)"=w315) -> (w316:T1)
                  }
                  frame Error {
                    n111 = local read "Current Position:"() -> (w319:dbl)
                  }
                }
              }
              frame "Grating Translation" {
                w333 = refnum<visa-resource-name> "COM8" ("VISA resource name IN")
                w334 = "D" ("Axis Prefix")
                n112 = call "AMS Move Motor.vi"("error in"=w335, "Motor steps"=-600000.0, "Axis Prefix"=w334, "VISA resource name IN"=w333) -> ("error out"=w336:errorcluster)  [unwired: 6 in, 1 out]
                n113 = Subtract(x=16160.0 ("Motor steps"), y=1800.0) -> (x-y=w324:dbl)
                n114 = call "AMS Move Motor.vi"("error in"=w336, "Motor steps"=w324, "Axis Prefix"=w334, "VISA resource name IN"=w333) -> ("error out"=w337:errorcluster)  [unwired: 6 in, 1 out]
                n115 = flat-sequence {
                  tunnel: [w346] -> w331
                  tunnel: w337 -> [w346]
                  frame #0 {
                    n116 = Wait (ms)(milliseconds to wait=u32 70000) -> ()  [unwired: 1 out]
                  }
                }
                n117 = case shown="No Error" w331 {
                  selector: w331 -> [w342 w345]
                  tunnel: [w342 w345] -> w330
                  tunnel: w329 -> [w341 w344]
                  tunnel: [w340 w344] -> w328
                  tunnel: [w339 w343] -> w327
                  frame No Error {
                    w339 = 0.0 ("Source Anode Rotation (P)")
                    n118 = Bundle By Name(cluster=w341, "Grating Translation (P)"=w339) -> (w340:T1)
                  }
                  frame Error {
                    n119 = local read "Current Position:"() -> (w343:dbl)
                  }
                }
              }
              frame "Grating Vertical" {
                w355 = refnum<visa-resource-name> "COM8" ("VISA resource name IN")
                w356 = "K" ("Axis Prefix")
                n120 = call "AMS Move Motor.vi"("error in"=w354, "Motor steps"=200000.0, "Axis Prefix"=w356, "VISA resource name IN"=w355) -> ("error out"=w357:errorcluster)  [unwired: 6 in, 1 out]
                n121 = call "AMS Move Motor.vi"("error in"=w357, "Motor steps"=-36590.0, "Axis Prefix"=w356, "VISA resource name IN"=w355) -> ("error out"=w358:errorcluster)  [unwired: 6 in, 1 out]
                n122 = flat-sequence {
                  tunnel: [w368] -> w348
                  tunnel: w358 -> [w368]
                  frame #0 {
                    n123 = Wait (ms)(milliseconds to wait=u32 70000) -> ()  [unwired: 1 out]
                  }
                }
                n124 = case shown="No Error" w348 {
                  selector: w348 -> [w361 w366]
                  tunnel: w351 -> [w364 w367]
                  tunnel: [w363 w367] -> w352
                  tunnel: [w362 w365] -> w350
                  tunnel: [w361 w366] -> w349
                  frame No Error {
                    w362 = 0.0 ("Source Anode Rotation (P)")
                    n125 = Bundle By Name(cluster=w364, "Grating Vertical (P)"=w362) -> (w363:T1)
                  }
                  frame Error {
                    n126 = local read "Current Position:"() -> (w365:dbl)
                  }
                }
              }
              frame "Grating Rotation" {
                w377 = refnum<visa-resource-name> "COM8" ("VISA resource name IN")
                w378 = "J" ("Axis Prefix")
                n127 = call "AMS Move Motor.vi"("error in"=w376, "Motor steps"=200000.0, "Axis Prefix"=w378, "VISA resource name IN"=w377) -> ("error out"=w379:errorcluster)  [unwired: 6 in, 1 out]
                n128 = call "AMS Move Motor.vi"("error in"=w379, "Motor steps"=-6280.0, "Axis Prefix"=w378, "VISA resource name IN"=w377) -> ("error out"=w380:errorcluster)  [unwired: 6 in, 1 out]
                n129 = flat-sequence {
                  tunnel: [w390] -> w374
                  tunnel: w380 -> [w390]
                  frame #0 {
                    n130 = Wait (ms)(milliseconds to wait=u32 30000) -> ()  [unwired: 1 out]
                  }
                }
                n131 = case shown="No Error" w374 {
                  selector: w374 -> [w386 w388]
                  tunnel: [w386 w388] -> w373
                  tunnel: w372 -> [w385 w387]
                  tunnel: [w384 w387] -> w371
                  tunnel: [w383 w389] -> w370
                  frame No Error {
                    w383 = 0.0 ("Source Anode Rotation (P)")
                    n132 = Bundle By Name(cluster=w385, "Grating Rotation (P)"=w383) -> (w384:T1)
                  }
                  frame Error {
                    n133 = local read "Current Position:"() -> (w389:dbl)
                  }
                }
              }
              frame "Polarization Angle" {
                n134 = One Button Dialog(message="No Home Position\nSet for this Axis.") -> ()  [unwired: 1 in, 1 out]
                n135 = local read "Current Position:"() -> (w393:dbl)
              }
              frame "Source Mirror Translation" {
                n136 = One Button Dialog(message="No Home Position\nSet for this Axis.") -> ()  [unwired: 1 in, 1 out]
                n137 = local read "Current Position:"() -> (w399:dbl)
              }
              frame "Source Mirror Rotation" {
                n138 = One Button Dialog(message="No Home Position\nSet for this Axis.") -> ()  [unwired: 1 in, 1 out]
                n139 = local read "Current Position:"() -> (w403:dbl)
              }
              frame "Camera Translation" {
                n140 = One Button Dialog(message="No Home Position\nSet for this Axis.") -> ()  [unwired: 1 in, 1 out]
                n141 = local read "Current Position:"() -> (w408:dbl)
              }
              frame "Camera Vertical" {
                n142 = One Button Dialog(message="No Home Position\nSet for this Axis.") -> ()  [unwired: 1 in, 1 out]
                n143 = local read "Current Position:"() -> (w413:dbl)
              }
              frame "Detector Mirror Rotation" {
                n144 = One Button Dialog(message="No Home Position\nSet for this Axis.") -> ()  [unwired: 1 in, 1 out]
                n145 = local read "Current Position:"() -> (w418:dbl)
              }
            }
            n146 = flat-sequence {
              tunnel: [w296] -> w287
              tunnel: w289 -> [w296]
              tunnel: w285 -> [w295]
              frame #0 {
                "Home" <- w295
              }
            }
            n147 = local write "Current Position:"(w286) -> ()
          }
          event "Reset Position to Target": Value Change {
            n148 = event-data() -> ()  [unwired: 1 in, 1 out]
            n149 = case shown="\"Camera Vertical\"" w429 {
              selector: w429 -> [w438 w465 w471 w476 w481 w485 w495 w498 w503 w508 w513]
              tunnel: w428 -> [w439 w466 w470 w475 w480 w486 w494 w500 w505 w510 w515]
              tunnel: "Target" -> [w435 w462 w467 w472 w477 w482 w488 w496 w501 w506 w511]
              tunnel: [w438 w465 w471 w476 w481 w485 w495 w498 w503 w508 w513] -> w426
              tunnel: [w436 w464 w469 w474 w479 w484 w493 w499 w504 w509 w514] -> w425
              tunnel: w422 -> [w437 w463 w468 w473 w478 w483 w492 w497 w502 w507 w512]
              tunnel: [w437 w463 w468 w473 w478 w483 w492 w497 w502 w507 w512] -> w424
              tunnel: [w433 w462 w467 w472 w477 w482 w488 w496 w501 w506 w511] -> w423
              frame "Source Anode Rotation", Default {
                n150 = case shown="0, Default" w435 {
                  tunnel: [0.0 ("Target") 0.0 ("Target") 468.0 ("Target") 936.0 ("Target") 1404.0 ("Target") 1872.0 ("Target") 2340.0 ("Target")] -> w433
                  tunnel: [u32 1 ("Anode :") u32 1 ("Anode :") u32 2 ("Anode :") u32 3 ("Anode :") u32 4 ("Anode :") u32 5 ("Anode :") u32 6 ("Anode :")] -> w434
                  tunnel: [enum16{"1", "2", "3", "4", "5", "6"}."1" ("Anode Control") enum16{"1", "2", "3", "4", "5", "6"}."1" ("Anode Control") enum16{"1", "2", "3", "4", "5", "6"}."2" ("Anode Control") enum16{"1", "2", "3", "4", "5", "6"}."3" ("Anode Control") enum16{"1", "2", "3", "4", "5", "6"}."4" ("Anode Control") enum16{"1", "2", "3", "4", "5", "6"}."5" ("Anode Control") enum16{"1", "2", "3", "4", "5", "6"}."6" ("Anode Control")] -> w432
                  frame 0, Default {
                    n151 = One Button Dialog(message="Enter 1-6 for Anode #") -> ()  [unwired: 1 in, 1 out]
                  }
                  frame 1 {
                  }
                  frame 2 {
                  }
                  frame 3 {
                  }
                  frame 4 {
                  }
                  frame 5 {
                  }
                  frame 6 {
                  }
                }
                n152 = local write "Anode :"(w434) -> ()
                n153 = local write "Anode Control"(w432) -> ()
                n154 = Bundle By Name(cluster=w439, "Source Anode Rotation (P)"=w433) -> (w436:T1)
              }
              frame "Aperture Translation" {
                n155 = Bundle By Name(cluster=w466, "Aperture Translation (P)"=w462) -> (w464:T1)
              }
              frame "Grating Translation" {
                n156 = Bundle By Name(cluster=w470, "Grating Translation (P)"=w467) -> (w469:T1)
              }
              frame "Grating Vertical" {
                n157 = Bundle By Name(cluster=w475, "Grating Vertical (P)"=w472) -> (w474:T1)
              }
              frame "Grating Rotation" {
                n158 = Bundle By Name(cluster=w480, "Grating Rotation (P)"=w477) -> (w479:T1)
              }
              frame "Polarization Angle" {
                n159 = Bundle By Name(cluster=w486, "Polarization Angle (P)"=w482) -> (w484:T1)
              }
              frame "Source Mirror Translation" {
                n160 = Bundle By Name(cluster=w494, "Source Mirror Translation (P)"=w488) -> (w493:T1)
                n161 = Subtract(x=3.7594, y=w488) -> (x-y=w490:dbl)
                n162 = Multiply(x=25.4, y=w490) -> (x*y=w487:dbl)
                n163 = local write "Source Mirror Position (mm)"(w487) -> ()
              }
              frame "Source Mirror Rotation" {
                n164 = Bundle By Name(cluster=w500, "Source Mirror Rotation (P)"=w496) -> (w499:T1)
              }
              frame "Camera Translation" {
                n165 = Bundle By Name(cluster=w505, "Camera Translation (P)"=w501) -> (w504:T1)
              }
              frame "Camera Vertical" {
                n166 = Bundle By Name(cluster=w510, "Camera Vertical (P)"=w506) -> (w509:T1)
              }
              frame "Detector Mirror Rotation" {
                n167 = Bundle By Name(cluster=w515, "Detector Mirror Rotation (P)"=w511) -> (w514:T1)
              }
            }
            n168 = local write "Current Position:"(w423) -> ()
          }
          event "Position Index +/-": Value Change {
            n169 = event-data() -> ()  [unwired: 1 in, 1 out]
            n170 = local read "Current Position:"() -> (w523:dbl)
            n171 = flat-sequence {
              tunnel: "Time Delay" -> [w534]
              tunnel: w520 -> [w533]
              tunnel: [w533] -> w519
              frame #0 {
                n172 = Multiply(x=w534, y=u32 1000) -> (x*y=w535:u32)
                n173 = Wait (ms)(milliseconds to wait=w535) -> ()  [unwired: 1 out]
              }
            }
            n174 = case shown="\"Aperture Translation\"" w527 {
              selector: w527 -> [w543 w567 w588 w609 w633 w650 w699 w730 w750 w772 w790]
              tunnel: w519 -> [w537 w563 w583 w603 w623 w645 w690 w719 w746 w768 w784]
              tunnel: [w540 w561 w581 w601 w625 w649 w683 w713 w744 w766 w788] -> w528
              tunnel: w521 -> [w545 w558 w589 w611 w632 w657 w698 w728 w741 w763 w791]
              tunnel: [w544 w557 w580 w610 w631 w656 w697 w729 w740 w762 w789] -> w526
              tunnel: [w543 w567 w588 w609 w633 w650 w699 w730 w750 w772 w790] -> w525
              tunnel: "Index +/- Value" -> [w538 w559 w579 w602 w624 w648 w692 w715 w742 w764 w785]
              tunnel: [w542 w566 w587 w608 w629 w658 w685 w727 w749 w771 w787] -> w517
              tunnel: w523 -> [w541 w560 w586 w607 w630 w647 w696 w726 w743 w765 w786]
              frame "Source Anode Rotation", Default {
                n175 = call "AMS Move Motor.vi"("error in"=w537, "Motor steps"=w538, "Axis Prefix"="M", "VISA resource name IN"=refnum<visa-resource-name> "COM8") -> ("error out"=w539:errorcluster)  [unwired: 6 in, 1 out]
                n176 = case shown="No Error" w539 {
                  selector: w539 -> [w549 w554]
                  tunnel: w545 -> [w553 w555]
                  tunnel: [w552 w555] -> w544
                  tunnel: [w551 w556] -> w542
                  tunnel: w541 -> [w550 w556]
                  tunnel: [w549 w554] -> w540
                  tunnel: w538 -> [w548 _]
                  frame No Error {
                    n177 = Add(x=w550, y=w548) -> (x+y=w551:dbl)
                    n178 = Bundle By Name(cluster=w553, "Source Anode Rotation (P)"=w551) -> (w552:T1)
                  }
                  frame Error {
                  }
                }
              }
              frame "Aperture Translation" {
                n179 = Multiply(x=w559, y=2000.0) -> (x*y=w565:dbl)
                n180 = call "AMS Move Motor.vi"("error in"=w563, "Motor steps"=w565, "Axis Prefix"="Z", "VISA resource name IN"=refnum<visa-resource-name> "COM8") -> ("error out"=w562:errorcluster)  [unwired: 6 in, 1 out]
                n181 = case shown="No Error" w562 {
                  selector: w562 -> [w574 w578]
                  tunnel: [w575 w576] -> w566
                  tunnel: [w574 w578] -> w561
                  tunnel: w560 -> [w573 w576]
                  tunnel: w559 -> [w572 _]
                  tunnel: w558 -> [w571 w577]
                  tunnel: [w570 w577] -> w557
                  frame No Error {
                    n182 = Add(x=w573, y=w572) -> (x+y=w575:dbl)
                    n183 = Bundle By Name(cluster=w571, "Aperture Translation (P)"=w575) -> (w570:T1)
                  }
                  frame Error {
                  }
                }
              }
              frame "Grating Translation" {
                n184 = Multiply(x=w579, y=2000.0) -> (x*y=w584:dbl)
                n185 = call "AMS Move Motor.vi"("error in"=w583, "Motor steps"=w584, "Axis Prefix"="D", "VISA resource name IN"=refnum<visa-resource-name> "COM8") -> ("error out"=w582:errorcluster)  [unwired: 6 in, 1 out]
                n186 = case shown="No Error" w582 {
                  selector: w582 -> [w594 w600]
                  tunnel: w589 -> [w597 w598]
                  tunnel: [w596 w599] -> w587
                  tunnel: w586 -> [w595 w599]
                  tunnel: [w594 w600] -> w581
                  tunnel: [w593 w598] -> w580
                  tunnel: w579 -> [w592 _]
                  frame No Error {
                    n187 = Add(x=w595, y=w592) -> (x+y=w596:dbl)
                    n188 = Bundle By Name(cluster=w597, "Grating Translation (P)"=w596) -> (w593:T1)
                  }
                  frame Error {
                  }
                }
              }
              frame "Grating Vertical" {
                n189 = Multiply(x=w602, y=2000.0) -> (x*y=w605:dbl)
                n190 = call "AMS Move Motor.vi"("error in"=w603, "Motor steps"=w605, "Axis Prefix"="K", "VISA resource name IN"=refnum<visa-resource-name> "COM8") -> ("error out"=w604:errorcluster)  [unwired: 6 in, 1 out]
                n191 = case shown="No Error" w604 {
                  selector: w604 -> [w614 w621]
                  tunnel: w611 -> [w619 w620]
                  tunnel: [w618 w620] -> w610
                  tunnel: [w617 w622] -> w608
                  tunnel: w607 -> [w616 w622]
                  tunnel: w602 -> [w615 _]
                  tunnel: [w614 w621] -> w601
                  frame No Error {
                    n192 = Add(x=w616, y=w615) -> (x+y=w617:dbl)
                    n193 = Bundle By Name(cluster=w619, "Grating Vertical (P)"=w617) -> (w618:T1)
                  }
                  frame Error {
                  }
                }
              }
              frame "Grating Rotation" {
                n194 = Multiply(x=w624, y=200.0) -> (x*y=w627:dbl)
                n195 = call "AMS Move Motor.vi"("error in"=w623, "Motor steps"=w627, "Axis Prefix"="B", "VISA resource name IN"=refnum<visa-resource-name> "COM8") -> ("error out"=w626:errorcluster)  [unwired: 6 in, 1 out]
                n196 = case shown="Error" w626 {
                  selector: w626 -> [w637 w642]
                  tunnel: w632 -> [w641 w644]
                  tunnel: [w640 w644] -> w631
                  tunnel: w630 -> [w639 w643]
                  tunnel: [w638 w643] -> w629
                  tunnel: [w637 w642] -> w625
                  tunnel: w624 -> [w636 _]
                  frame No Error {
                    n197 = Add(x=w639, y=w636) -> (x+y=w638:dbl)
                    n198 = Bundle By Name(cluster=w641, "Grating Rotation (P)"=w638) -> (w640:T1)
                  }
                  frame Error {
                  }
                }
              }
              frame "Polarization Angle" {
                # "^   Limits of Polarization angle \n      due to table interference"
                n199 = Add(x=w648, y=w647) -> (x+y=w655:dbl)
                n200 = Greater Or Equal?(x=130.0, y=w655) -> (x >= y?=w651:bool)
                n201 = Greater Or Equal?(x=w655, y=-95.0) -> (x >= y?=w652:bool)
                n202 = And(x=w651, y=w652) -> (x .and. y?=w646:bool)
                n203 = case shown="True" w646 {
                  tunnel: [w659 w675] -> w658
                  tunnel: w648 -> [_ w665]
                  tunnel: w647 -> [w659 w667]
                  tunnel: w657 -> [w662 w674]
                  tunnel: [w662 w673] -> w656
                  tunnel: w645 -> [w661 w668]
                  tunnel: [w661 w668] -> w649
                  frame False {
                    n204 = One Button Dialog(message="Polarization Angle Out of Range.\n\nPlease enter a different value.\nMax  = 130\nMin  = -35") -> ()  [unwired: 1 in, 1 out]
                  }
                  frame True {
                    n205 = Greater Or Equal To 0?(x=w665) -> (x >= 0?=w666:bool)
                    n206 = case shown="True" w666 {
                      tunnel: w665 -> [w677 w681]
                      tunnel: [w678 w680] -> w664
                      tunnel: 3.0 ("y") -> [w676 w679]
                      frame False {
                        n207 = Subtract(x=w677, y=w676) -> (x-y=w678:dbl)
                      }
                      frame True {
                        n208 = Add(x=w681, y=w679) -> (x+y=w680:dbl)
                      }
                    }
                    n209 = call "polarmotor_DAQmxNoCheck.vi"("Position (Deg) 2"=w667, "Num Degrees"=w664, "Free"=FALSE, "Free2"=FALSE, "Speed"=FALSE, "C-on"=TRUE) -> ()  [unwired: 4 in, 2 out]
                    n210 = Add(x=w667, y=w665) -> (x+y=w675:dbl)
                    n211 = Bundle By Name(cluster=w674, "Polarization Angle (P)"=w675) -> (w673:T1)
                  }
                }
              }
              frame "Source Mirror Translation" {
                n212 = Divide(x=w692, y=25.4) -> (x/y=w682:dbl)
                n213 = Multiply(x=w682, y=512000.0 ("x")) -> (x*y=w687:dbl)
                n214 = Format Into String(format string="%d", w687) -> (resulting string=w693:string)  [unwired: 2 in, 1 out]
                n215 = call "MDrive_Set_Parameter_dual_axis.vi"("Axis"=Axis."Translation", "error in"=w690, "Parameter Setpoint"=w693, "Set Parameter"=Set_Parameter."Move Relative (MR)", "VISA resource name in"=refnum<visa-resource-name> "COM6" ("VISA resource name")) -> ("error out"=w684:errorcluster)  [unwired: 2 in, 1 out]
                n216 = case shown="No Error" w684 {
                  selector: w684 -> [w702 w711]
                  tunnel: w698 -> [w709 w710]
                  tunnel: [w708 w710] -> w697
                  tunnel: w696 -> [w701 w712]
                  tunnel: [w706 w712] -> w685
                  tunnel: [w702 w711] -> w683
                  tunnel: w682 -> [w700 _]
                  frame No Error {
                    n217 = Subtract(x=w701, y=w700) -> (x-y=w706:dbl)
                    n218 = Subtract(x=3.7594, y=w706) -> (x-y=w705:dbl)
                    n219 = Multiply(x=25.4, y=w705) -> (x*y=→"Source Mirror Position (mm)":dbl)
                    n220 = Bundle By Name(cluster=w709, "Source Mirror Translation (P)"=w706) -> (w708:T1)
                  }
                  frame Error {
                  }
                }
              }
              frame "Source Mirror Rotation" {
                n221 = Divide(x=w715, y=-3.75) -> (x/y=w723:dbl)
                n222 = Multiply(x=51200.0, y=w723) -> (x*y=w722:dbl)
                n223 = Format Into String(format string="%d", w722) -> (resulting string=w718:string)  [unwired: 2 in, 1 out]
                n224 = call "MDrive_Set_Parameter_dual_axis.vi"("Axis"=Axis."Rotation", "error in"=w719, "Parameter Setpoint"=w718, "Set Parameter"=Set_Parameter."Move Relative (MR)", "VISA resource name in"=refnum<visa-resource-name> "COM6" ("VISA resource name")) -> ("error out"=w714:errorcluster)  [unwired: 2 in, 1 out]
                n225 = case shown="No Error" w714 {
                  selector: w714 -> [w731 w737]
                  tunnel: [w736 w738] -> w729
                  tunnel: w728 -> [w735 w738]
                  tunnel: [w734 w739] -> w727
                  tunnel: w726 -> [w733 w739]
                  tunnel: w715 -> [w732 _]
                  tunnel: [w731 w737] -> w713
                  frame No Error {
                    n226 = Add(x=w733, y=w732) -> (x+y=w734:dbl)
                    n227 = Bundle By Name(cluster=w735, "Source Mirror Rotation (P)"=w734) -> (w736:T1)
                  }
                  frame Error {
                  }
                }
              }
              frame "Camera Translation" {
                n228 = Multiply(x=w742, y=2000.0) -> (x*y=w748:dbl)
                n229 = call "AMS Move Motor.vi"("error in"=w746, "Motor steps"=w748, "Axis Prefix"="C", "VISA resource name IN"=refnum<visa-resource-name> "COM8") -> ("error out"=w745:errorcluster)  [unwired: 6 in, 1 out]
                n230 = case shown="No Error" w745 {
                  selector: w745 -> [w757 w761]
                  tunnel: [w758 w759] -> w749
                  tunnel: [w757 w761] -> w744
                  tunnel: w743 -> [w756 w759]
                  tunnel: w742 -> [w755 _]
                  tunnel: w741 -> [w754 w760]
                  tunnel: [w753 w760] -> w740
                  frame No Error {
                    n231 = Add(x=w756, y=w755) -> (x+y=w758:dbl)
                    n232 = Bundle By Name(cluster=w754, "Camera Translation (P)"=w758) -> (w753:T1)
                  }
                  frame Error {
                  }
                }
              }
              frame "Camera Vertical" {
                n233 = Multiply(x=w764, y=2000.0) -> (x*y=w770:dbl)
                n234 = call "AMS Move Motor.vi"("error in"=w768, "Motor steps"=w770, "Axis Prefix"="P", "VISA resource name IN"=refnum<visa-resource-name> "COM8") -> ("error out"=w767:errorcluster)  [unwired: 6 in, 1 out]
                n235 = case shown="No Error" w767 {
                  selector: w767 -> [w779 w783]
                  tunnel: [w780 w781] -> w771
                  tunnel: [w779 w783] -> w766
                  tunnel: w765 -> [w778 w781]
                  tunnel: w764 -> [w777 _]
                  tunnel: w763 -> [w776 w782]
                  tunnel: [w775 w782] -> w762
                  frame No Error {
                    n236 = Add(x=w778, y=w777) -> (x+y=w780:dbl)
                    n237 = Bundle By Name(cluster=w776, "Camera Vertical (P)"=w780) -> (w775:T1)
                  }
                  frame Error {
                  }
                }
              }
              frame "Detector Mirror Rotation" {
                w798 = 1.0  # Steps/degree
                n238 = Multiply(x=w785, y=w798) -> (x*y=w792:dbl)
                n239 = call "SMC_INIT.vi"("error in (no error)"=w784, "SMC Parameter"=T9 {"VENUS Language"=enum."VENUS 2", "Number of Axis"=1, "Controller Nr"=1, "Simulation"=FALSE}, "Communication Parameter"=T7 {"Comm Method"=enum."VISA", "IP Address"="", "Remote Port"=23, "GPIB Address"="", "VISA Resource Name"="COM1", "Visa Baud Rate"=19200, "Visa Serial"=TRUE}) -> ("error out"=w794:errorcluster)  [unwired: 8 in]
                n240 = call "SMC_AxisRel.vi"("error in (no error)"=w794, "WaitUntilReady"=TRUE, "Distance"=w792, "AxisNr"=u8 1) -> ("error out"=w793:errorcluster)  [unwired: 7 in]
                n241 = case shown="No Error" w793 {
                  selector: w793 -> [w804 w808]
                  tunnel: [w806 w809] -> w789
                  tunnel: w791 -> [w805 w809]
                  tunnel: [w803 w807] -> w787
                  tunnel: w786 -> [w802 w807]
                  tunnel: [w804 w808] -> w797
                  tunnel: w785 -> [w801 _]
                  frame No Error {
                    n242 = Add(x=w802, y=w801) -> (x+y=w803:dbl)
                    n243 = Bundle By Name(cluster=w805, "Detector Mirror Rotation (P)"=w803) -> (w806:T1)
                  }
                  frame Error {
                  }
                }
                n244 = call "SMC_Close.vi"("error in (no error)"=w797) -> ("error out"=w788:errorcluster)  [unwired: 10 in]
              }
            }
            n245 = Equal To 0?(x=w517) -> (x = 0?=w516:bool)
            n246 = local write "Current Position:"(w517) -> ()
            n247 = case shown="False" w516 {
              selector: w516 -> [w531 w532]
              frame False {
                n248 = local write "Home"(w531) -> ()
              }
              frame True {
                n249 = local write "Home"(w532) -> ()
              }
            }
            n250 = local write "Home"(FALSE) -> ()
          }
          event "Move to Absolute Positon": Value Change {
            n251 = event-data() -> ()  [unwired: 1 in, 1 out]
            n252 = local read "Current Position:"() -> (w818:dbl)
            n253 = local read "Time Delay"() -> (w812:u32)
            n254 = flat-sequence {
              tunnel: w812 -> [w827]
              tunnel: [w826] -> w814
              tunnel: w813 -> [w826]
              frame #0 {
                n255 = Multiply(x=w827, y=u32 1000) -> (x*y=w828:u32)
                n256 = Wait (ms)(milliseconds to wait=w828) -> ()  [unwired: 1 out]
              }
            }
            n257 = case shown="\"Camera Vertical\"" w819 {
              tunnel: "Absolute Position Value" -> [_ _ _ _ _ _ w857 _ _ _ _]
              tunnel: w814 -> [w833 w837 w841 w845 w849 w853 w865 w887 w891 w895 w899]
              tunnel: [w833 w837 w841 w845 w849 w853 w861 w887 w891 w895 w899] -> w820
              tunnel: w818 -> [w831 w835 w839 w843 w847 w851 w859 w885 w889 w893 w897]
              tunnel: w817 -> [w832 w836 w840 w844 w848 w852 w864 w886 w890 w894 w898]
              tunnel: [w832 w836 w840 w844 w848 w852 w863 w886 w890 w894 w898] -> w816
              tunnel: [w831 w835 w839 w843 w847 w851 w860 w885 w889 w893 w897] -> w810
              frame "Source Anode Rotation", Default {
                n258 = One Button Dialog(message="Absolute positioning is not \navailable for this axis.") -> ()  [unwired: 1 in, 1 out]
              }
              frame "Aperture Translation" {
                n259 = One Button Dialog(message="Absolute positioning is not \navailable for this axis.") -> ()  [unwired: 1 in, 1 out]
              }
              frame "Grating Translation" {
                n260 = One Button Dialog(message="Absolute positioning is not \navailable for this axis.") -> ()  [unwired: 1 in, 1 out]
              }
              frame "Grating Vertical" {
                n261 = One Button Dialog(message="Absolute positioning is not \navailable for this axis.") -> ()  [unwired: 1 in, 1 out]
              }
              frame "Grating Rotation" {
                n262 = One Button Dialog(message="Absolute positioning is not \navailable for this axis.") -> ()  [unwired: 1 in, 1 out]
              }
              frame "Polarization Angle" {
                n263 = One Button Dialog(message="Absolute positioning is not \navailable for this axis.") -> ()  [unwired: 1 in, 1 out]
              }
              frame "Source Mirror Translation" {
                n264 = local read "Source Mirror Position (mm)"() -> (w858:dbl)
                n265 = Subtract(x=w857, y=w858) -> (x-y=w855:dbl)
                n266 = Divide(x=w855, y=25.4) -> (x/y=w856:dbl)
                n267 = Multiply(x=w856, y=512000.0 ("x")) -> (x*y=w866:dbl)
                n268 = Format Into String(format string="%d", w866) -> (resulting string=w870:string)  [unwired: 2 in, 1 out]
                n269 = call "MDrive_Set_Parameter_dual_axis.vi"("Axis"=Axis."Translation", "error in"=w865, "Parameter Setpoint"=w870, "Set Parameter"=Set_Parameter."Move Relative (MR)", "VISA resource name in"=refnum<visa-resource-name> "COM6" ("VISA resource name")) -> ("error out"=w862:errorcluster)  [unwired: 2 in, 1 out]
                n270 = case shown="No Error" w862 {
                  selector: w862 -> [w878 w883]
                  tunnel: w864 -> [w880 w882]
                  tunnel: [w879 w882] -> w863
                  tunnel: [w878 w883] -> w861
                  tunnel: [w873 w881] -> w860
                  tunnel: w859 -> [_ w881]
                  tunnel: w857 -> [w875 _]
                  frame No Error {
                    n271 = Divide(x=w875, y=25.4) -> (x/y=w874:dbl)
                    n272 = local write "Source Mirror Position (mm)"(w875) -> ()
                    n273 = Subtract(x=3.7594 ("y"), y=w874) -> (x-y=w873:dbl)
                    n274 = Bundle By Name(cluster=w880, "Source Mirror Translation (P)"=w873) -> (w879:T1)
                  }
                  frame Error {
                  }
                }
              }
              frame "Source Mirror Rotation" {
                n275 = One Button Dialog(message="Absolute positioning is not \navailable for this axis.") -> ()  [unwired: 1 in, 1 out]
              }
              frame "Camera Translation" {
                n276 = One Button Dialog(message="Absolute positioning is not \navailable for this axis.") -> ()  [unwired: 1 in, 1 out]
              }
              frame "Camera Vertical" {
                n277 = One Button Dialog(message="Absolute positioning is not \navailable for this axis.") -> ()  [unwired: 1 in, 1 out]
              }
              frame "Detector Mirror Rotation" {
                n278 = One Button Dialog(message="Absolute positioning is not \navailable for this axis.") -> ()  [unwired: 1 in, 1 out]
              }
            }
            n279 = Equal To 0?(x=w810) -> (x = 0?=w811:bool)
            n280 = local write "Current Position:"(w810) -> ()
            n281 = case shown="True" w811 {
              selector: w811 -> [w824 w825]
              frame False {
                n282 = local write "Home"(w824) -> ()
              }
              frame True {
                n283 = local write "Home"(w825) -> ()
              }
            }
            n284 = local write "Home"(FALSE) -> ()
          }
          event "Stop Motion Softly": Value Change {
            n285 = event-data() -> ()  [unwired: 1 in, 1 out]
            n286 = case shown="\"Camera Vertical\"" w906 {
              selector: w906 -> [w909 w915 w921 w927 w933 w940 w944 w948 w951 w957 w964]
              tunnel: w900 -> [w911 w917 w923 w929 w935 w941 w945 w949 w953 w959 w965]
              tunnel: [w910 w916 w922 w928 w934 w941 w945 w949 w952 w958 w965] -> w905
              tunnel: [w909 w915 w921 w927 w933 w940 w944 w948 w951 w957 w964] -> w903
              tunnel: [w908 w914 w920 w926 w932 w939 w943 w947 w950 w956 w963] -> w901
              tunnel: w902 -> [w908 w914 w920 w926 w932 w939 w943 w947 w950 w956 w963]
              frame "Source Anode Rotation", Default {
                n287 = call "AMS Stop Motor.vi"("error in"=w911, "Axis Prefix"="M", "VISA resource name IN"=refnum<visa-resource-name> "COM8") -> ("error out"=w910:errorcluster)  [unwired: 7 in, 1 out]
              }
              frame "Aperture Translation" {
                n288 = call "AMS Stop Motor.vi"("error in"=w917, "Axis Prefix"="G", "VISA resource name IN"=refnum<visa-resource-name> "COM8") -> ("error out"=w916:errorcluster)  [unwired: 7 in, 1 out]
              }
              frame "Grating Translation" {
                n289 = call "AMS Stop Motor.vi"("error in"=w923, "Axis Prefix"="D", "VISA resource name IN"=refnum<visa-resource-name> "COM8") -> ("error out"=w922:errorcluster)  [unwired: 7 in, 1 out]
              }
              frame "Grating Vertical" {
                n290 = call "AMS Stop Motor.vi"("error in"=w929, "Axis Prefix"="K", "VISA resource name IN"=refnum<visa-resource-name> "COM8") -> ("error out"=w928:errorcluster)  [unwired: 7 in, 1 out]
              }
              frame "Grating Rotation" {
                n291 = call "AMS Stop Motor.vi"("error in"=w935, "Axis Prefix"="J", "VISA resource name IN"=refnum<visa-resource-name> "COM8") -> ("error out"=w934:errorcluster)  [unwired: 7 in, 1 out]
              }
              frame "Polarization Angle" {
                n292 = One Button Dialog(message="Stop function not available \nfor this axis.") -> ()  [unwired: 1 in, 1 out]
              }
              frame "Source Mirror Translation" {
                n293 = One Button Dialog(message="Stop function not available \nfor this axis.") -> ()  [unwired: 1 in, 1 out]
              }
              frame "Source Mirror Rotation" {
                n294 = One Button Dialog(message="Stop function not available \nfor this axis.") -> ()  [unwired: 1 in, 1 out]
              }
              frame "Camera Translation" {
                n295 = call "AMS Stop Motor.vi"("error in"=w953, "Axis Prefix"="C", "VISA resource name IN"=refnum<visa-resource-name> "COM8") -> ("error out"=w952:errorcluster)  [unwired: 7 in, 1 out]
              }
              frame "Camera Vertical" {
                n296 = call "AMS Stop Motor.vi"("error in"=w959, "Axis Prefix"="P", "VISA resource name IN"=refnum<visa-resource-name> "COM8") -> ("error out"=w958:errorcluster)  [unwired: 7 in, 1 out]
              }
              frame "Detector Mirror Rotation" {
                n297 = One Button Dialog(message="Stop function not available \nfor this axis.") -> ()  [unwired: 1 in, 1 out]
              }
            }
          }
          event "Anode Control": Value Change {
            # "468 Motor Steps \nbetween each \nanode position"
            n298 = event-data() -> ()  [unwired: 1 in, 1 out]
            n299 = Unbundle By Name(w972) -> ("Source Anode Rotation (P)"=w978:dbl)
            n300 = case shown="\"4\"" "Anode Control" {
              tunnel: w978 -> [w985 w996 w1002 w1009 w1017 w1025]
              tunnel: [w982 w994 w1000 w1008 w1016 w1024] -> w975
              tunnel: [u32 1 ("Anode :") u32 2 ("Anode :") u32 3 ("Anode :") u32 4 ("Anode :") u32 5 ("Anode :") u32 6 ("Anode :")] -> w974
              tunnel: 468.0 ("y") -> [w984 w992 w1004 w1010 w1018 w1026]
              tunnel: w972 -> [w988 w993 w999 w1007 w1015 w1023]
              tunnel: [w988 w993 w999 w1007 w1015 w1023] -> w971
              tunnel: [w983 w990 w998 w1006 w1014 w1022] -> w966
              frame "1", Default {
                n301 = Multiply(x=0.0, y=w984) -> (x*y=w983:dbl)
                n302 = Subtract(x=w985, y=w983) -> (x-y=w987:dbl)
                n303 = Negate(x=w987) -> (-x=w982:dbl)
              }
              frame "2" {
                n304 = Multiply(x=1.0, y=w992) -> (x*y=w990:dbl)
                n305 = Subtract(x=w996, y=w990) -> (x-y=w995:dbl)
                n306 = Negate(x=w995) -> (-x=w994:dbl)
              }
              frame "3" {
                n307 = Multiply(x=2.0, y=w1004) -> (x*y=w998:dbl)
                n308 = Subtract(x=w1002, y=w998) -> (x-y=w1001:dbl)
                n309 = Negate(x=w1001) -> (-x=w1000:dbl)
              }
              frame "4" {
                n310 = Multiply(x=3.0, y=w1010) -> (x*y=w1006:dbl)
                n311 = Subtract(x=w1009, y=w1006) -> (x-y=w1011:dbl)
                n312 = Negate(x=w1011) -> (-x=w1008:dbl)
              }
              frame "5" {
                n313 = Multiply(x=4.0, y=w1018) -> (x*y=w1014:dbl)
                n314 = Subtract(x=w1017, y=w1014) -> (x-y=w1019:dbl)
                n315 = Negate(x=w1019) -> (-x=w1016:dbl)
              }
              frame "6" {
                n316 = Multiply(x=5.0, y=w1026) -> (x*y=w1022:dbl)
                n317 = Subtract(x=w1025, y=w1022) -> (x-y=w1027:dbl)
                n318 = Negate(x=w1027) -> (-x=w1024:dbl)
              }
            }
            "Anode :" <- w974
            n319 = Bundle By Name(cluster=w971, "Source Anode Rotation (P)"=w966) -> (w970:T1)
            n320 = call "AMS Move Motor.vi"("error in"=w968, "Motor steps"=w975, "Axis Prefix"="M", "VISA resource name IN"=refnum<visa-resource-name> "COM8") -> ("error out"=w969:errorcluster)  [unwired: 6 in, 1 out]
          }
          event "Abort Motion": Value Change {
            n321 = event-data() -> ()  [unwired: 1 in, 1 out]
            n322 = One Button Dialog(message="Not Available") -> ()  [unwired: 1 in, 1 out]
          }
          event "Source Voltage Control": Value Change {
            n323 = event-data() -> ()  [unwired: 1 in, 1 out]
            n324 = local read "Logging Indicator"() -> (w1041:bool)
            n325 = Not(x=w1041) -> (.not. x?=w1040:bool)
            n326 = case shown="True" w1040 {
              selector: w1040 -> [w1044 _]
              tunnel: [w1044 w1046] -> w1039
              frame False {
                w1045 = T11."Disabled and Grayed Out" ("Disabled")
                n327 = property on="Source Voltage" class="DigNum (strict)"("DisabledEnum"=w1045) -> ()  [unwired: 2 in, 2 out]
                n328 = property on="Current (mA)" class="DigNum (strict)"("DisabledEnum"=w1045) -> ()  [unwired: 2 in, 2 out]
                n329 = property on="Set Source Voltage" class="Bool"("DisabledEnum"=w1045) -> ()  [unwired: 2 in, 2 out]
                n330 = property on="Voltage Value" class="DigNum (strict)"("DisabledEnum"=w1045) -> ()  [unwired: 2 in, 2 out]
              }
              frame True {
                n331 = Two Button Dialog(message="Only click \"Continue\" if High\nVoltage supply on source \nrack is turned ON.", 2:"Continue" ("T button name (\"OK\")")) -> (T button?=w1048:bool)  [unwired: 1 in]
                n332 = case shown="True" w1048 {
                  selector: w1048 -> [w1050 w1051]
                  tunnel: [w1050 w1051] -> w1046
                  frame False {
                  }
                  frame True {
                    w1052 = T11."Enabled" ("Disabled")
                    n333 = property on="Source Voltage" class="DigNum (strict)"("DisabledEnum"=w1052) -> ()  [unwired: 2 in, 2 out]
                    n334 = property on="Current (mA)" class="DigNum (strict)"("DisabledEnum"=w1052) -> ()  [unwired: 2 in, 2 out]
                    n335 = property on="Set Source Voltage" class="Bool"("DisabledEnum"=w1052) -> ()  [unwired: 2 in, 2 out]
                    n336 = property on="Voltage Value" class="DigNum (strict)"("DisabledEnum"=w1052) -> ()  [unwired: 2 in, 2 out]
                  }
                }
              }
            }
            "Logging Indicator" <- w1039
          }
          event "Set Source Voltage": Value Change {
            n337 = event-data() -> ()  [unwired: 1 in, 1 out]
            n338 = local read "Logging Indicator"() -> (w1056:bool)
            n339 = case shown="True" w1056 {
              frame False {
              }
              frame True {
                n340 = call "SetVoltage.vi"("Voltage"="Voltage Value", "Address"=u16 3) -> ()  [unwired: 10 out]
              }
            }
          }
        }
      }
      frame "Add New State Here" {
      }
    }
    n341 = Unbundle By Name(w69) -> ("status"=→"Error":bool)
    n342 = local write "Axis Positions"(w71) -> ()
  }
  n343 = call <vilib>:"Simple Error Handler.vi"("error in (no error)"=w3) -> ()  [unwired: 4 in, 5 out]
  n344 = while {
    tunnel: 1000 -> [w1066]
    stop <- w1067 stop-if-true
    n345 = event shown="[0] Timeout" {
      selector: _ -> [_ _]
      dyn-events: _ -> [_ _]
      timeout: w1066 -> [_ _]
      tunnel: [FALSE TRUE] -> w1067
      event Timeout {
        # "When setup, use\nAIN2 for diode 3"
        n346 = event-data() -> ()  [unwired: 1 in, 1 out]
        n347 = local read "Logging Indicator"() -> (w1075:bool)
        n348 = case shown="False" w1075 {
          frame False {
          }
          frame True {
            w1082 = u16 0 items=["Voltage and Current", "Voltage Only", "Current Only"] ("Measure")
            n349 = call "ReadVoltage.vi"("Measure"=w1082, "Address"=i16 3) -> ("Current"=w1080:dbl, "Voltage"=→"Source Voltage":dbl)
            n350 = Multiply(x=w1080, y=1000.0) -> (x*y=→"Current (mA)":dbl)
          }
        }
        n351 = call "U3 eAIN Read Diode Voltage.vi"("Channel-P"=0) -> ("Output Voltage"=w1071:dbl)  [unwired: 9 in, 1 out]
        n352 = call "U3 eAIN Read Diode Voltage.vi"("Channel-P"=1) -> ("Output Voltage"=w1069:dbl)  [unwired: 9 in, 1 out]
        n353 = Number To Fractional String(number=w1071, precision (6)=i16 2) -> (F-format string=→"Diode 2":string)  [unwired: 2 in]
        n354 = Number To Fractional String(number=w1069, precision (6)=i16 2) -> (F-format string=→"Diode 1":string)  [unwired: 2 in]
      }
      event "Stop Program": Value Change {
        n355 = event-data() -> ()  [unwired: 1 in, 1 out]
      }
    }
  }
  n356 = flat-sequence {
    tunnel: w9 -> [w1086]
    frame #0 {
      n357 = local write "Error"(FALSE) -> ()
      n358 = call <vilib>:"Simple Error Handler.vi"("error in (no error)"=w1086) -> ()  [unwired: 4 in, 5 out]
    }
  }
